vi "cara.vi"() -> ()   [LabVIEW 2016]
panel:
  out "new picture":picture
  in  "Horizontal Pointer Slide":dbl(slide) scale=0.0..255.0
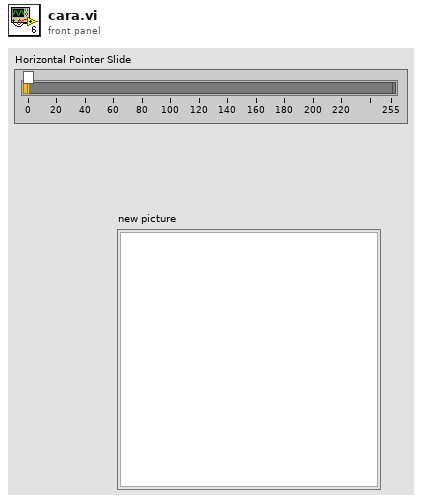
[diagram p1: front panel]
types:
  T1 = typedef "imagedata.ctl" = cluster{"image type":i32, "image depth":i32, "image":u8[], "mask":u8[], "colors":u32[], "Rectangle":cluster{"left":i16, "top":i16, "right":i16, "bottom":i16}}
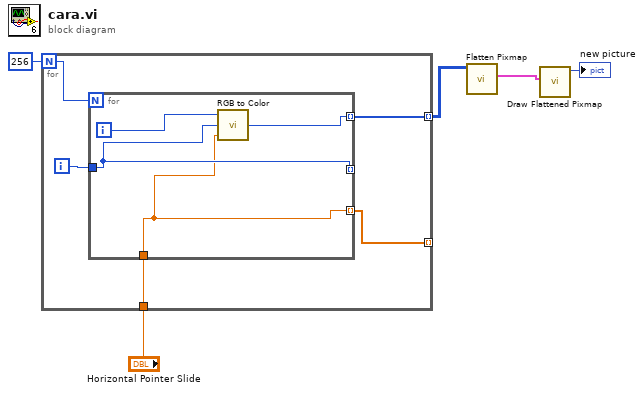
[diagram p0: block diagram]
diagram:
  n1 = for {
    N: 256 -> [w10]
    tunnel: [w8] -> _ mode=indexing
    tunnel: [w7] -> w4 mode=indexing
    tunnel: "Horizontal Pointer Slide" -> [w6]
    i -> [w9]
    n2 = for {
      N: w10 -> [_]
      tunnel: w9 -> [w14]
      tunnel: [w12] -> w8 mode=indexing
      tunnel: [w14] -> _ mode=indexing
      tunnel: [w11] -> w7 mode=indexing
      tunnel: w6 -> [w12]
      i -> [w13]
      n3 = call <vilib>:"RGB to Color.vi"("B"=w12, "G"=w14, "R"=w13) -> ("Color"=w11:u32)
    }
  }
  n4 = call <vilib>:"Flatten Pixmap.vi"("24-bit pixmap"=w4) -> ("image data"=w2:T1)  [unwired: 10 in]
  n5 = call <vilib>:"Draw Flattened Pixmap.vi"("image data"=w2) -> ("new picture"=→"new picture":picture)  [unwired: 8 in]
